vi "Write write operation timeout.vi"(8 "error in (no error)":errorcluster, 10 "write operation timeout":u32=100, 11 "SMSD ADU in":refnum<class "SMSD ADU.lvclass">) -> (0 "error out":errorcluster, 3 "SMSD ADU out":refnum<class "SMSD ADU.lvclass">)   [LabVIEW 2021, in "SMSD ADU.lvclass"]
uses:
  SMSD ADU.lvclass
  SMSD ADU.lvclass/SMSD ADU.ctl
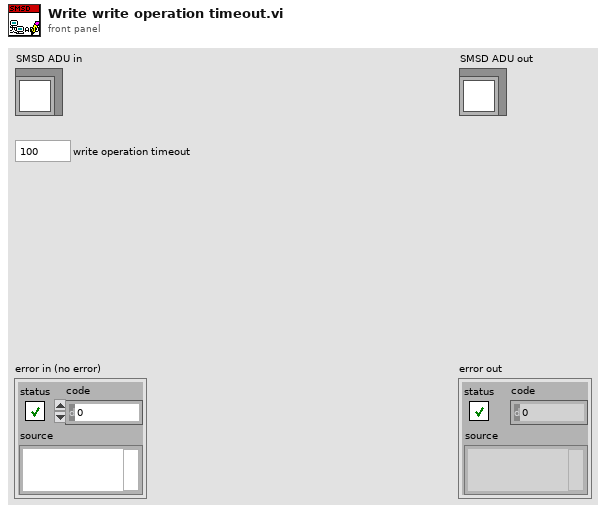
[diagram p1: front panel]
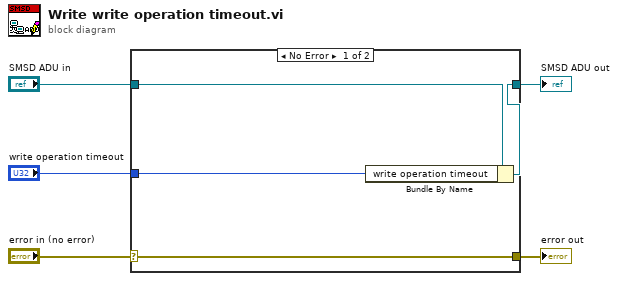
[diagram p0: block diagram]
diagram:
  n1 = case shown="No Error" "error in (no error)" {
    selector: "error in (no error)" -> [w9 w10]
    tunnel: [w9 w10] -> w4
    tunnel: [w7 w11] -> w2
    tunnel: "SMSD ADU in" -> [w8 w11]
    tunnel: "write operation timeout" -> [w6 _]
    frame No Error {
      n2 = Bundle By Name(cluster=w8, "write operation timeout"=w6) -> (w7:refnum<class "SMSD ADU.lvclass">)
    }
    frame Error {
    }
  }
  "error out" <- w4
  "SMSD ADU out" <- w2
